vi "Sort Reverse Alphabetical.vi"(0 "Unsorted Array":string[](array[string]), 11 "Error In":errorcluster) -> (4 "Sorted Array":string[](array[string]), 15 "Error Out":errorcluster)   [LabVIEW 2019, in "File and Path Operations.lvlib"]
doc: "This VI sorts an array of strings in reverse alphabetical order (Z to A). It returns the sorted array or the default array in case of an error."
uses:
  File and Path Operations.lvlib
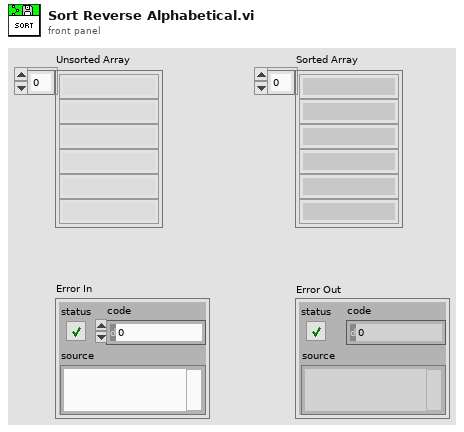
[diagram p1: front panel]
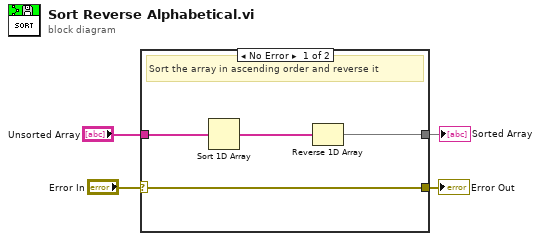
[diagram p0: block diagram]
diagram:
  n1 = case shown="No Error" "Error In" {
    selector: "Error In" -> [w8 w9]
    tunnel: [w8 w9] -> w3
    tunnel: [w5 _] -> w1
    tunnel: "Unsorted Array" -> [w7 _]
    frame No Error {
      # "Sort the array in ascending order and reverse it"
      n2 = Sort 1D Array(array=w7) -> (sorted array=w6:string[])
      n3 = Reverse 1D Array(array=w6) -> (reversed array=w5:string[])
    }
    frame Error {
      # "Returns the default value"
    }
  }
  "Error Out" <- w3
  "Sorted Array" <- w1
